vi "Sandbox VI 1.vi"() -> ()   [LabVIEW 2016]
doc: "The first bold characters are: 22, 23, 24, 25"
uses:
  <vilib>/Utility/traverseref.llb/TRef TravTarget.ctl
  <vilib>/Utility/traverseref.llb/VI Scripting - Traverse.lvlib
panel:
  out "Font:Bold 22-30":bool
  out "Font:Bold 22-27":bool
  out "Font:Bold 22-26":bool
  out "Font:Bold 21-25":bool
  out "Font:Bold 22-25":bool
  out "Font:Bold 22-23":bool
  out "Font:Bold 3":bool
  out "Array":bool[](array[boolean])
  out "Iteration 2":i32
  out "Font:Bold 2":bool
  out "Font:Bold":bool
  out "Text":string
  out "Text":string
  out "Iteration":i32
  out "error out":errorcluster
  out "# of Refs":i32
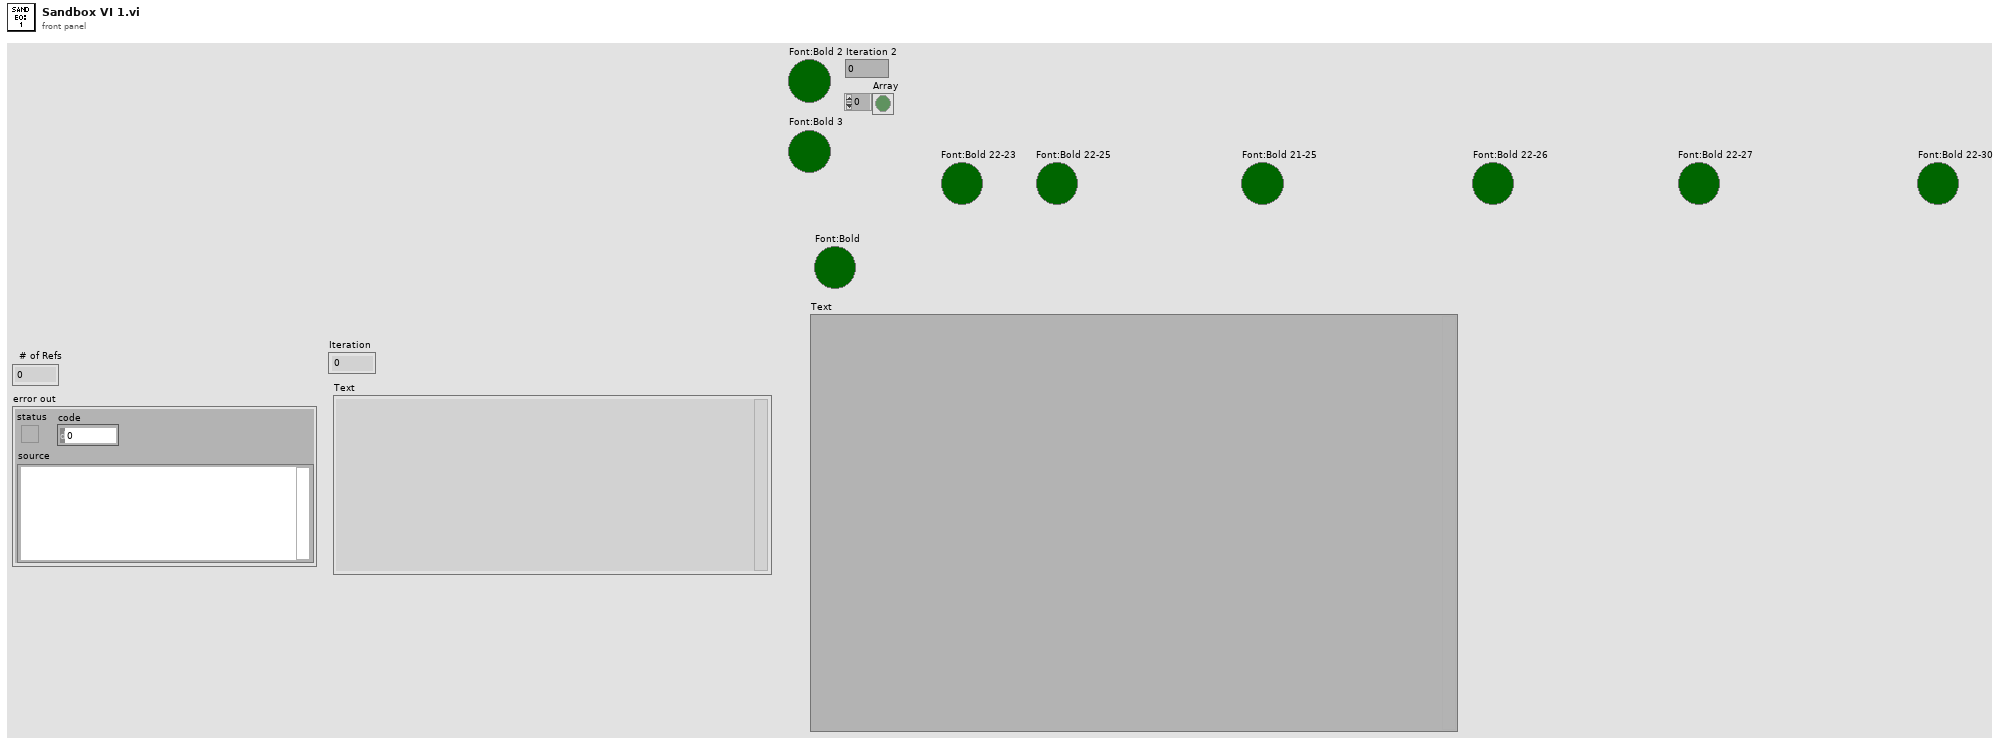
[diagram p1: front panel]
types:
  T1 = typedef "TRef TravTarget.ctl" = enum16{"FP", "BD", "Other"}
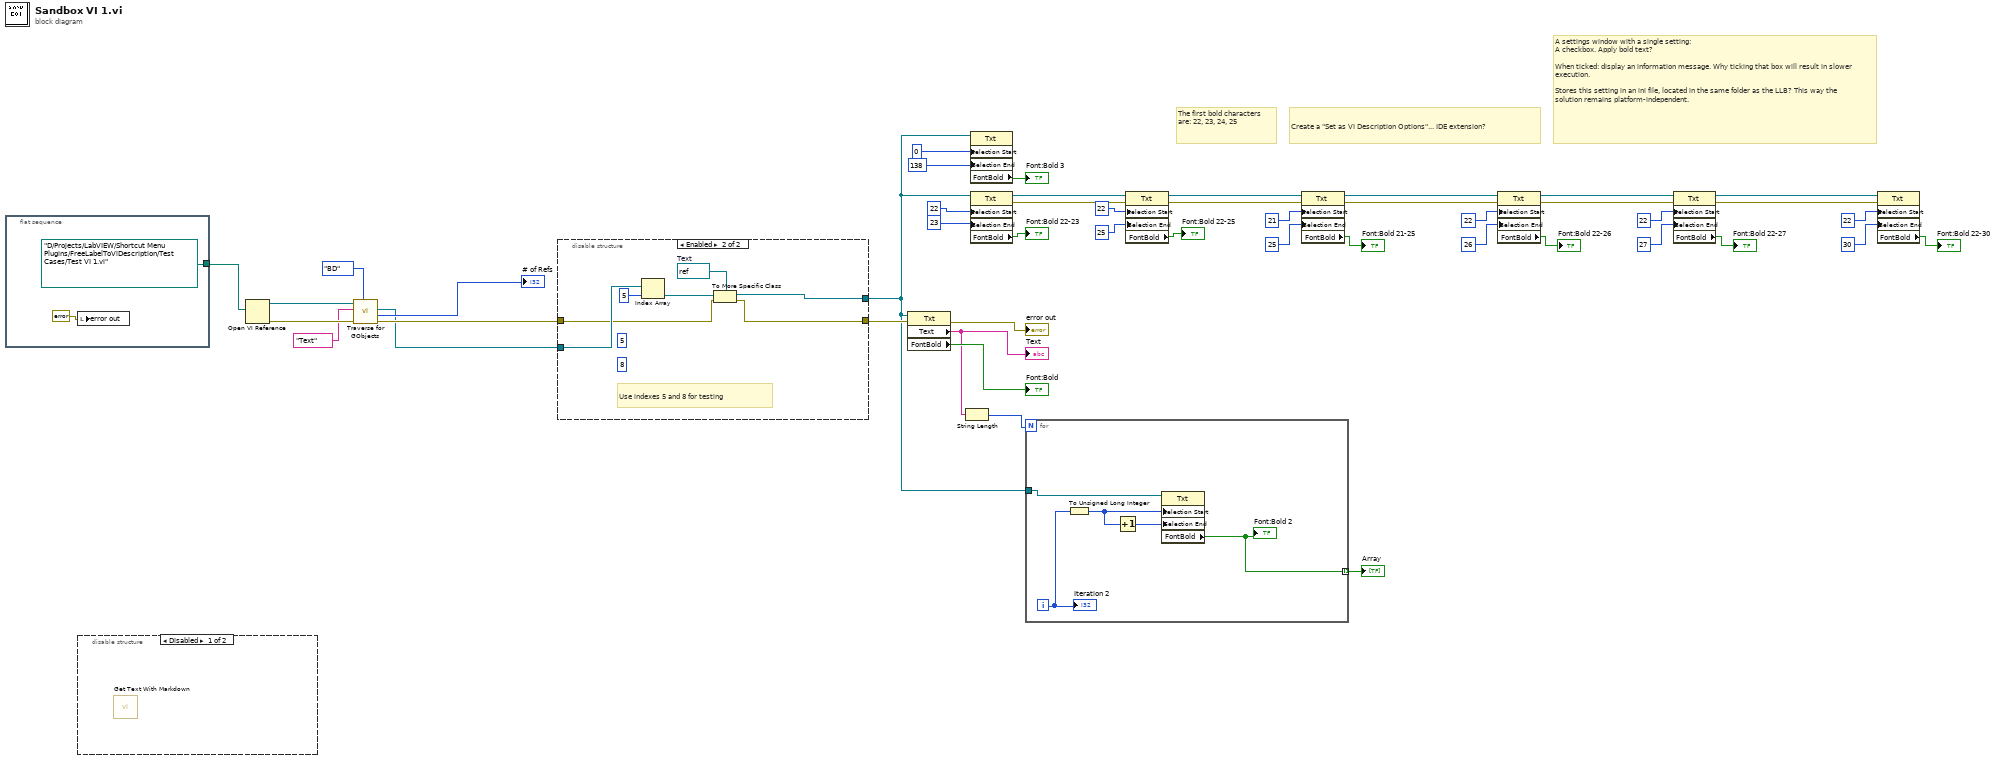
[diagram p0: block diagram]
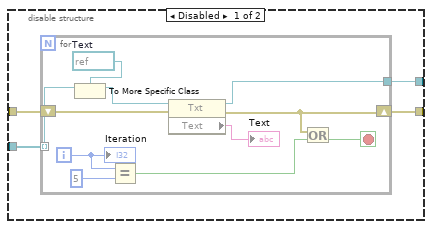
[diagram p2: hidden frame]
diagram:
  # "A settings window with a single setting:\nA checkbox. Apply bold text?\n\nWhen ticked: display an information message. Why ticking that box will result in slower execution.\n\nStores this setting in an ini file, located in the same folder as the LLB? This way the solution remains platform-independent."
  # "Create a \"Set as VI Description Options\"... IDE extension?"
  # "The first bold characters are: 22, 23, 24, 25"
  n1 = flat-sequence {
    tunnel: [path "D:/Projects/LabVIEW/Shortcut Menu Plugins/FreeLabelToViDescription/Test Cases/Test VI 1.vi"] -> w46
    frame #0 {
      n2 = local write "error out"(errorcluster {"status"=FALSE, "code"=0, "source"=""} ("error in (no error)")) -> ()
    }
  }
  n3 = disable-structure shown="Disabled" {
    frame Disabled {
      n4 = call "Get Text With Markdown.vi"() -> ()  [unwired: 8 in, 4 out]
    }
    frame Enabled {
    }
  }
  n5 = Open VI Reference(vi path=w46) -> (vi reference=w44:refnum<vi>, error out=w45:errorcluster)  [unwired: 5 in]
  n6 = call <vilib>:"Traverse for GObjects.vi"("Traverse Target"=TRef_TravTarget."BD", "error in (no error)"=w45, "Class Name"="Text", "VI Refnum"=w44) -> ("error out"=w40:errorcluster, "# of Refs"=→"# of Refs":i32, "References"=w39:refnum<vi>[])  [unwired: 4 in, 1 out]
  n7 = disable-structure shown="Enabled" {
    disable-tunnel: w40 -> [w52 w67]
    disable-tunnel: [w51 w66] -> w38
    disable-tunnel: w39 -> [w50 w68]
    disable-tunnel: [w49 w64] -> w26
    frame Disabled {
      n8 = for {
        tunnel: w50 -> [w63] mode=indexing
        shift-right: [w58] -> w51
        shift-left: w52 -> [w60]
        tunnel: [w57] -> w49
        i -> [w55]
        stop <- w56 stop-if-true
        w61 = refnum<vi> refnum  # Text
        n9 = To More Specific Class(target class=w61, reference=w63) -> (specific class reference=w62:refnum<vi>)  [unwired: 1 in, 1 out]
        n10 = Equal?(x=w55, y=5) -> (x = y?=w53:bool)
        n11 = property class="Txt"(reference=w62, error in=w60) -> (reference out=w57:refnum<vi>, error out=w58:errorcluster, "Text"=→"Text":string)
        n12 = Or(x=w58, y=w53) -> (x .or. y?=w56:bool)
        "Iteration" <- w55
      }
    }
    frame Enabled {
      (unwired) 8 ("index")
      (unwired) 5 ("index")
      w65 = refnum<vi> refnum  # Text
      # "Use indexes 5 and 8 for testing"
      n13 = Index Array(array=w68, index=5) -> (element=w70:refnum<vi>)
      n14 = To More Specific Class(target class=w65, reference=w70, error in=w67) -> (specific class reference=w64:refnum<vi>, error out=w66:errorcluster)
    }
  }
  n15 = property class="Txt"(reference=w26, error in=w38) -> (error out=→"error out":errorcluster, "Text"=w35:string, "FontBold"=→"Font:Bold":bool)  [unwired: 1 out]
  "Text" <- w35
  n16 = String Length(string=w35) -> (length=w34:i32)
  n17 = property class="Txt"(reference=w26, "Selection Start"=u32 0 ("Selection:Start"), "Selection End"=u32 138 ("Selection:Start")) -> ("FontBold"=→"Font:Bold 3":bool)  [unwired: 1 in, 2 out]
  n18 = property class="Txt"(reference=w26, "Selection Start"=u32 22 ("Selection:Start"), "Selection End"=u32 23 ("Selection:Start")) -> (reference out=w24:refnum<vi>, error out=w23:errorcluster, "FontBold"=→"Font:Bold 22-23":bool)  [unwired: 1 in]
  n19 = for {
    N: w34 -> [_]
    tunnel: w26 -> [w75]
    tunnel: [w71] -> w33 mode=indexing
    i -> [w74]
    n20 = To Unsigned Long Integer(number=w74) -> (unsigned 32bit integer=w72:u32)
    n21 = Increment(x=w72) -> (x+1=w73:u32)
    n22 = property class="Txt"(reference=w75, "Selection Start"=w72, "Selection End"=w73) -> ("FontBold"=w71:bool)  [unwired: 1 in, 2 out]
    "Font:Bold 2" <- w71
    "Iteration 2" <- w74
  }
  "Array" <- w33
  n23 = property class="Txt"(reference=w24, error in=w23, "Selection Start"=u32 22 ("Selection:Start"), "Selection End"=u32 25 ("Selection:Start")) -> (reference out=w17:refnum<vi>, error out=w16:errorcluster, "FontBold"=→"Font:Bold 22-25":bool)
  n24 = property class="Txt"(reference=w17, error in=w16, "Selection Start"=u32 21 ("Selection:Start"), "Selection End"=u32 25 ("Selection:Start")) -> (reference out=w11:refnum<vi>, error out=w12:errorcluster, "FontBold"=→"Font:Bold 21-25":bool)
  n25 = property class="Txt"(reference=w11, error in=w12, "Selection Start"=u32 22 ("Selection:Start"), "Selection End"=u32 26 ("Selection:Start")) -> (reference out=w7:refnum<vi>, error out=w6:errorcluster, "FontBold"=→"Font:Bold 22-26":bool)
  n26 = property class="Txt"(reference=w7, error in=w6, "Selection Start"=u32 22 ("Selection:Start"), "Selection End"=u32 27 ("Selection:Start")) -> (reference out=w1:refnum<vi>, error out=w2:errorcluster, "FontBold"=→"Font:Bold 22-27":bool)
  n27 = property class="Txt"(reference=w1, error in=w2, "Selection Start"=u32 22 ("Selection:Start"), "Selection End"=u32 30 ("Selection:Start")) -> ("FontBold"=→"Font:Bold 22-30":bool)  [unwired: 2 out]
